vi "Continuous Receive with Send.vi"() -> ()   [LabVIEW 2014, in "GEA2_Toolkit.lvlib"]
uses:
  library/GEA2_Toolkit.lvlib
  type defs/Data Out.ctl
  type defs/Data In.ctl
  Washer HCC/Washer HCC NEWFI/LabVIEW GEA2 Toolkit/LabVIEW_GEA2_Toolkit.lvlibp
panel:
  in  "Input Data":T1={"Source"=228, "Destination"=0, "Command"=0, "Message"=""} {"Command" format="%02x"; "Destination" format="%02x"; "Source" format="%02x"}
  in  "Stop":bool
  out "Data Out":T2[](array[typedef]) {"CRC" format="%04x"; "Length" format="%02x"; "Command" format="%02x"; "Destination" format="%02x"; "Source" format="%02x"}
  in  "Send":bool
  out "Error Out":errorcluster
  in  "Error In":errorcluster
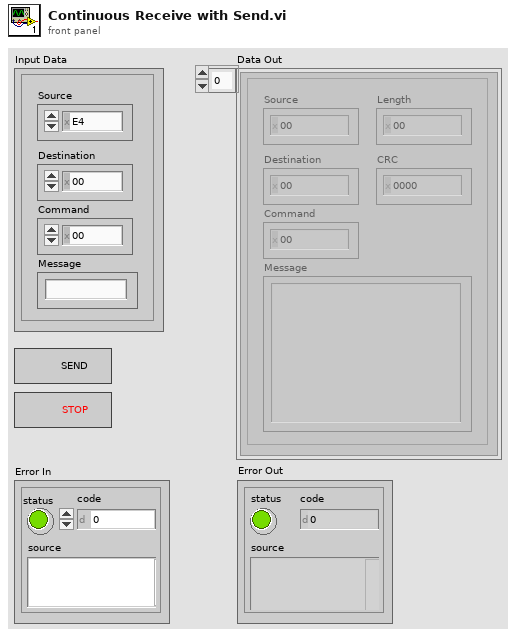
[diagram p1: front panel]
types:
  T1 = typedef "GEA2_Toolkit.lvlib/Data In.ctl" = cluster{"Source":u8, "Destination":u8, "Command":u8, "Message":string}
  T2 = typedef "GEA2_Toolkit.lvlib/Data Out.ctl" = cluster{"Source":u8, "Destination":u8, "Command":u8, "Length":u8, "CRC":u16, "Message":string}
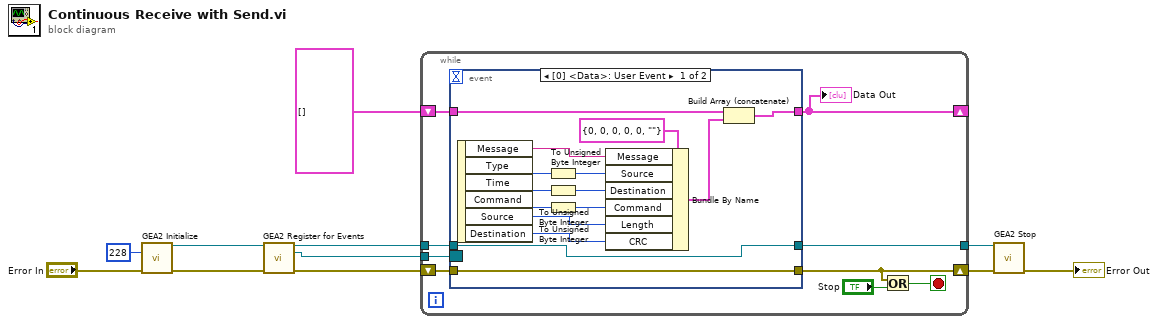
[diagram p0: block diagram]
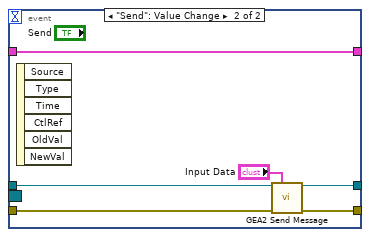
[diagram p2: hidden frame]
diagram:
  n1 = call "GEA2 Initialize.vi"("Source Address"=u8 228, "error in"="Error In") -> ("GEA2 Reference Out"=w9:refnum<k24>, "error out"=w10:errorcluster)  [unwired: 11 in, 1 out]
  n2 = call "GEA2 Register for Events.vi"("GEA2 Reference In"=w9, "Error In"=w10) -> ("GEA2 Reference Out"=w4:refnum<k24>, "GEA2 Event Registration"=w2:refnum<event-registration>, "Error Out"=w3:errorcluster)  [unwired: 11 in]
  n3 = while {
    tunnel: w2 -> [w18]
    tunnel: [w15] -> w7
    tunnel: w4 -> [w16]
    shift-right: [w14] -> w6
    shift-left: w3 -> [w17]
    shift-right: [w12] -> _
    shift-left: T2[] [] -> [w13]
    stop <- w19 stop-if-true
    n4 = event shown="[0] <Data>: User Event" {
      selector: w18 -> [_ _]
      dyn-events: _ -> [_ _]
      timeout: _ -> [_ _]
      tunnel: w17 -> [w35 w39]
      tunnel: [w35 w38] -> w14
      tunnel: w16 -> [w21 w41]
      tunnel: [w21 w40] -> w15
      tunnel: w13 -> [w24 w36]
      tunnel: [w22 w36] -> w12
      event User Event {
        n5 = event-data() -> ("Message"=w25:string, "Type"=w28:u32, "Time"=w29:u32, "Command"=w30:u8, "Source"=w27:u8, "Destination"=w26:u8)  [unwired: 1 in]
        n6 = To Unsigned Byte Integer(number=w28) -> (unsigned 8bit integer=w32:u8)
        n7 = To Unsigned Byte Integer(number=w29) -> (unsigned 8bit integer=w33:u8)
        n8 = To Unsigned Byte Integer(number=w30) -> (unsigned 8bit integer=w31:u8)
        n9 = Bundle By Name(cluster=T2 {"Source"=0, "Destination"=0, "Command"=0, "Length"=0, "CRC"=0, "Message"=""} ("Coverted Data Out"), "Message"=w25, "Source"=w32, "Destination"=w33, "Command"=w31, "Length"=w27, "CRC"=w26) -> (w23:T2)
        n10 = Build Array (concatenate)(w24, w23) -> (w22:T2[])
      }
      event "Send": Value Change {
        n11 = event-data() -> ()  [unwired: 1 in, 6 out]
        n12 = call "GEA2 Send Message.vi"("GEA2 Reference In"=w41, "Input Data"="Input Data", "Error In"=w39) -> ("GEA2 Reference Out"=w40:refnum<k24>, "Error Out"=w38:errorcluster)  [unwired: 11 in]
      }
    }
    "Data Out" <- w12
    n13 = Or(x=w14, y="Stop") -> (x .or. y?=w19:bool)
  }
  n14 = call "GEA2 Stop.vi"("GEA2 Reference In"=w7, "Error In"=w6) -> ("Error Out"=→"Error Out":errorcluster)  [unwired: 13 in]
